vi "Generate DocMap.vi"(10 "Array 2":T2[](array[typedef]), 11 "Array":T1[](array[typedef])) -> (3 "Variant":variant)   [LabVIEW 2017]
uses:
  _Typedef/DocNote.ctl
  _Typedef/DocElement.ctl
  csmdoc.lvlib
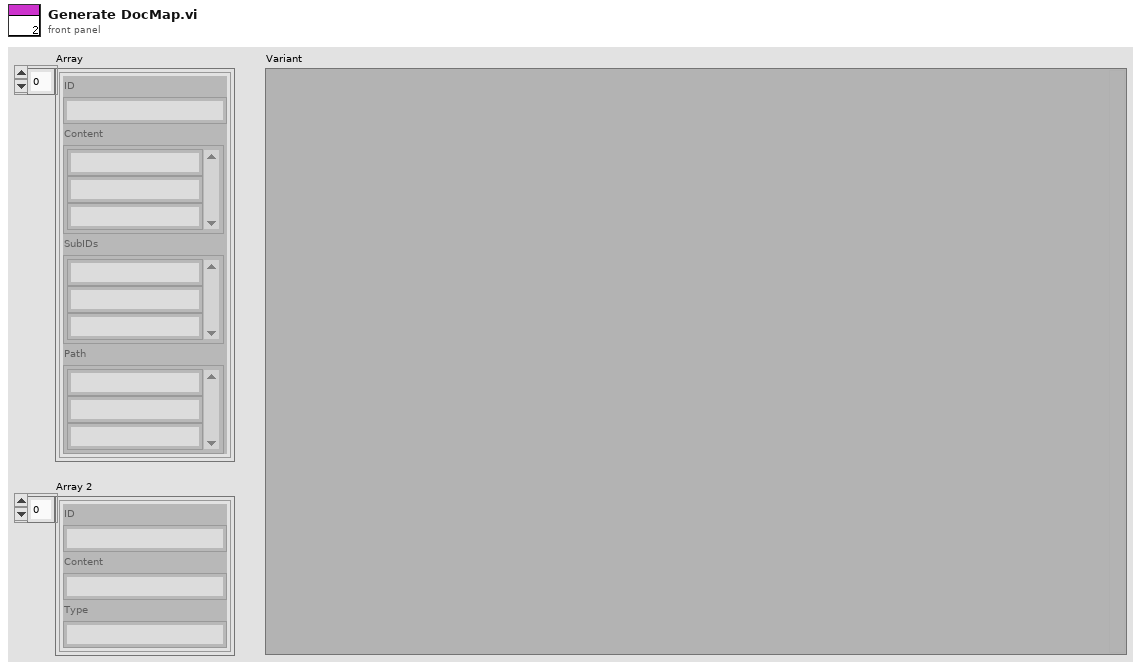
[diagram p1: front panel]
types:
  T1 = typedef "csmdoc.lvlib/DocElement.ctl" = cluster{"ID":string, "Content":string[], "SubIDs":string[], "Path":string[]}
  T2 = typedef "csmdoc.lvlib/DocNote.ctl" = cluster{"ID":string, "Content":string, "Type":string}
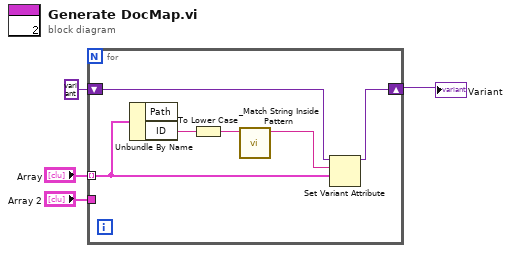
[diagram p0: block diagram]
diagram:
  n1 = for {
    tunnel: "Array" -> [w10] mode=indexing
    shift-right: [w8] -> w3
    shift-left: variant -> [w9]
    tunnel: "Array 2" -> [_]
    n2 = Unbundle By Name(w10) -> ("ID"=w7:string)  [unwired: 1 out]
    n3 = To Lower Case(string=w7) -> (all lower case string=w6:string)
    n4 = call "_Match String Inside Pattern.vi"("string"=w6) -> ("String inside"=w5:string)  [unwired: 10 in]
    n5 = Set Variant Attribute(Variant=w9, name=w5, value=w10) -> (Variant out=w8:variant)  [unwired: 1 in, 2 out]
  }
  "Variant" <- w3
